vi "Obtain.vi"(7 "max queue size (-1, unlimited)":i32=-1, 8 "error in (no error)":errorcluster, 9 "create if not found? (T)":bool=TRUE, 10 "Name (\"\")":string, 11 "Queue in":refnum<class "Queue.lvclass">) -> (0 "error out":errorcluster, 1 "created new?(T)":bool, 3 "Queue out":refnum<class "Queue.lvclass">)   [LabVIEW 2020, in "Data.lvlib" / "Queue.lvclass"]
doc: "Obtain a data queue."
uses:
  Queue.lvclass
  Data.lvclass
  Queue.lvclass/Queue.ctl
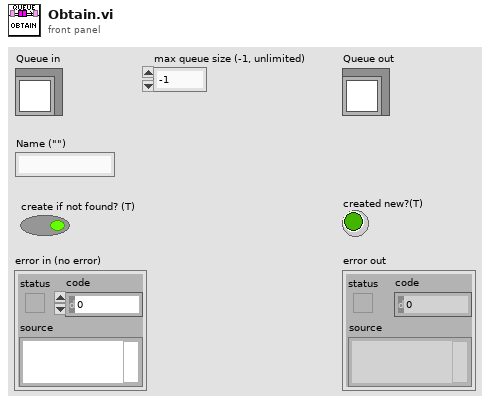
[diagram p1: front panel]
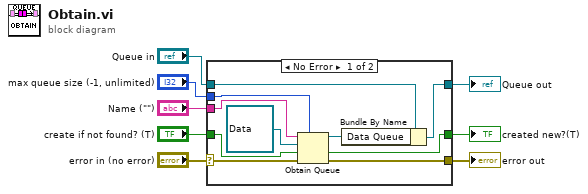
[diagram p0: block diagram]
diagram:
  n1 = case shown="No Error" "error in (no error)" {
    selector: "error in (no error)" -> [w11 w20]
    tunnel: [w10 w20] -> w7
    tunnel: [w17 w19] -> w5
    tunnel: "Queue in" -> [w18 w19]
    tunnel: "Name (\"\")" -> [w14 _]
    tunnel: "create if not found? (T)" -> [w13 _]
    tunnel: [w12 _] -> w2
    tunnel: "max queue size (-1, unlimited)" -> [w9 _]
    frame No Error {
      n2 = Obtain Queue(max queue size (-1, unlimited)=w9, name (unnamed)=w14, element data type=refnum<class "Data.lvclass"> refnum ("Data.lvlib:Data.lvclass"), create if not found? (T)=w13, error in (no error)=w11) -> (queue out=w16:refnum<queue>, created new?=w12:bool, error out=w10:errorcluster)
      n3 = Bundle By Name(cluster=w18, "Data Queue"=w16) -> (w17:refnum<class "Queue.lvclass">)
    }
    frame Error {
    }
  }
  "error out" <- w7
  "Queue out" <- w5
  "created new?(T)" <- w2
